vi "Compiled.Get Monitor Tool Settings.vi"(8 "error in (no error)":errorcluster, 9 "Database Ref":refnum<k21>, 11 "Addon Ref":T1 format="%.0x") -> (0 "error out":errorcluster, 2 "MonitorToolSettings":T2 {"Command Refs"."Response Refs"."Block Data Refs" format="%.0x"; "Command Refs"."Command Refs"."Block Data Refs"."Data Reference" format="%.0x"; "Data"."IncomingDataRefs"."Data Reference" format="%.0x"; "Data"."OutgoingDataRefs"."Data Reference" format="%.0x"; "Network"."Name" format="%.0x"}, 3 "Addon Ref out":T1 format="%.0x")   [LabVIEW 2015, in "J1939 Addon System Explorer.lvlib"]
uses:
  J1939 Addon System Explorer.lvlib
  <vilib>/NI Veristand/Custom Device API/Custom Device Item Ref.ctl
  Shared/Types/Compiled Monitor Tool Settings.ctl
  Shared/Types/Monitor Settings.ctl
  Shared/Types/Device Settings.ctl
  <vilib>/NI Veristand/Custom Device API/Block Data Reference.ctl
  <vilib>/NI Veristand/Custom Device API/Data Reference.ctl
  Shared/Types/Frame Settings.ctl
  Shared/Types/SysDef Command Settings.ctl
  <vilib>/NI Veristand/Custom Device Tools/Custom Device Utility Library/NI VeriStand - Search for Item by GUID.vi
  Shared/SubVIs/Constants.vi
  <vilib>/NI Veristand/Custom Device Tools/Custom Device Utility Library/Custom Device Utility Library.lvlib
  Shared/J1939 Addon Shared.lvlib
  <vilib>/NI VeriStand/Custom Device API/Custom Device API.lvlib
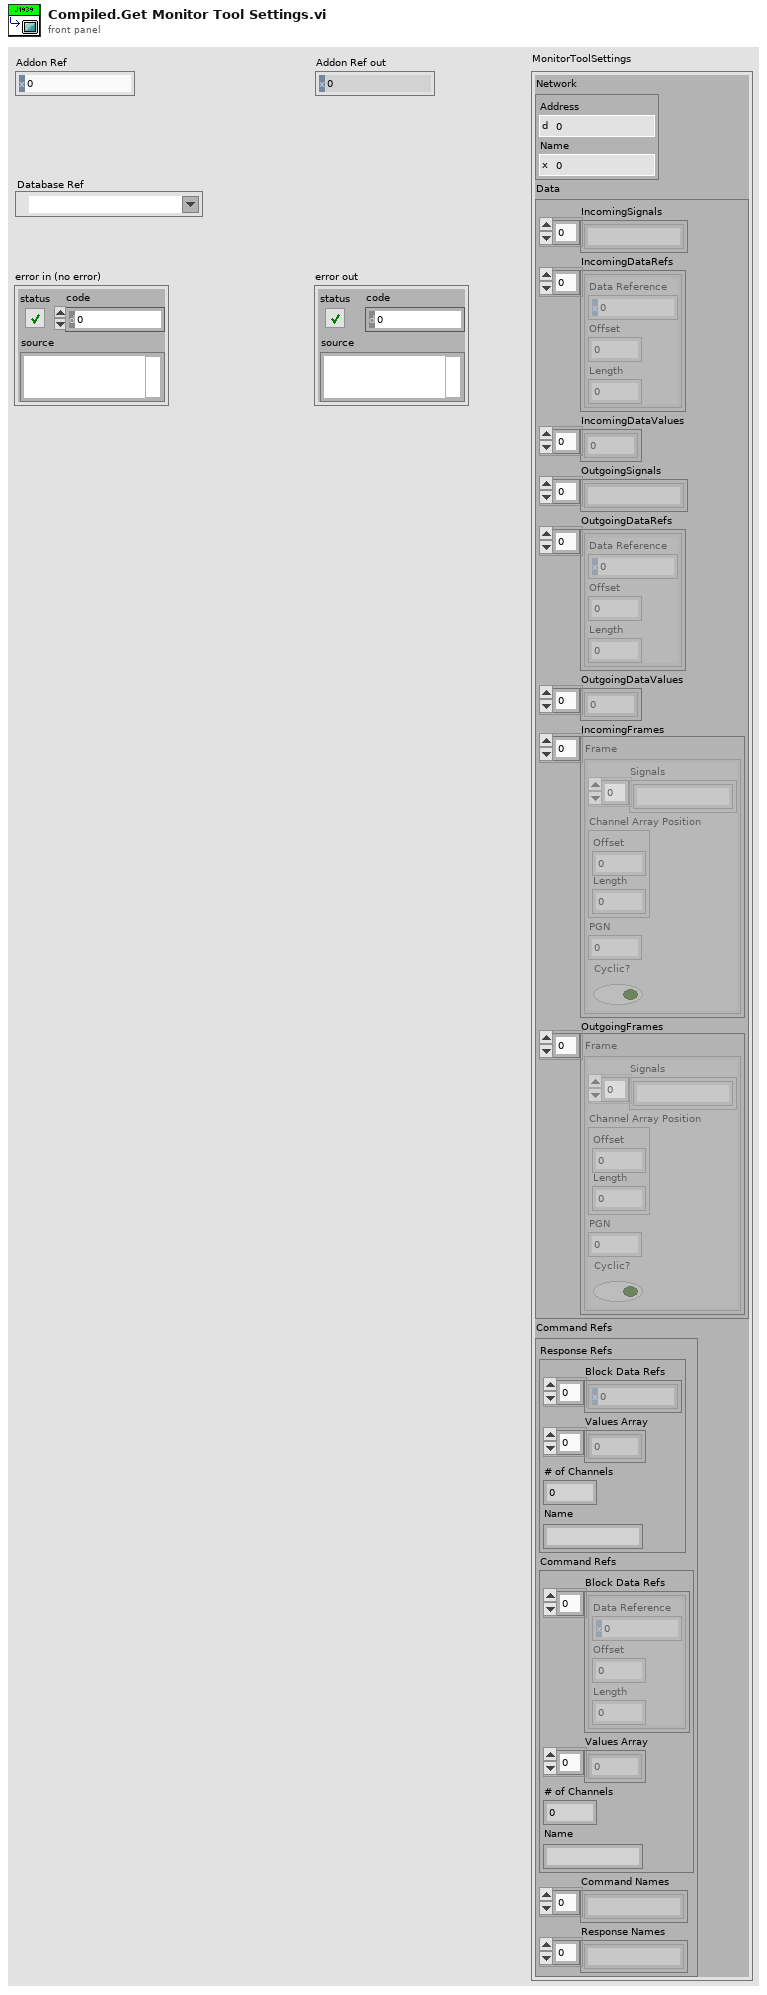
[diagram p1: front panel]
types:
  T1 = typedef "Custom Device API.lvlib/Custom Device Item Ref.ctl" = u64
  T2 = typedef "J1939 Addon Shared.lvlib/Compiled Monitor Tool Settings.ctl" = cluster{"Network":T3, "Data":T4, "Command Refs":T8}
  T3 = typedef "J1939 Addon Shared.lvlib/Monitor Settings.ctl" = cluster{"Address":u8, "Name":u64}
  T4 = typedef "J1939 Addon Shared.lvlib/Device Settings.ctl" = cluster{"IncomingSignals":string[], "IncomingDataRefs":T5[], "IncomingDataValues":dbl[], "OutgoingSignals":string[], "OutgoingDataRefs":T5[], "OutgoingDataValues":dbl[], "IncomingFrames":T7[], "OutgoingFrames":T7[]}
  T5 = typedef "Custom Device API.lvlib/Block Data Reference.ctl" = cluster{"Data Reference":T6, "Offset":u64, "Length":u64}
  T6 = typedef "Custom Device API.lvlib/Data Reference.ctl" = i32
  T7 = typedef "J1939 Addon Shared.lvlib/Frame Settings.ctl" = cluster{"Signals":string[], "Channel Array Position":cluster{"Offset":u32, "Length":u32}, "PGN":u32, "Cyclic?":bool}
  T8 = typedef "J1939 Addon Shared.lvlib/SysDef Command Settings.ctl" = cluster{"Response Refs":cluster{"Block Data Refs":T6[], "Values Array":dbl[], "# of Channels":u32, "Name":string}, "Command Refs":cluster{"Block Data Refs":T5[], "Values Array":dbl[], "# of Channels":u32, "Name":string}, "Command Names":string[], "Response Names":string[]}
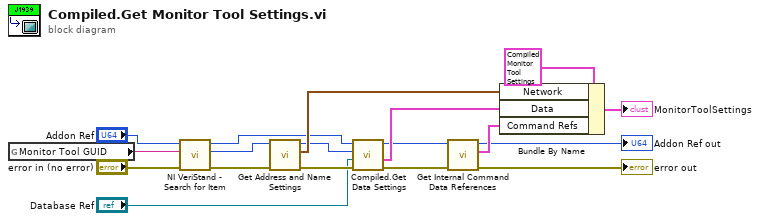
[diagram p0: block diagram]
diagram:
  n1 = global read "Constants.vi" "Monitor Tool GUID"() -> (w7:string)
  n2 = call-poly <vilib>:"NI VeriStand - Search for Item.vi"("error in"="error in (no error)", "Item GUID"=w7, "Section Ref in"="Addon Ref") -> ("error out"=w14:errorcluster, "Item Ref"=w15:T1, "Section Ref out"=w6:T1)  [unwired: 5 in, 1 out]
  n3 = call "Get Address and Name Settings.vi"("error in (no error)"=w14, "Node Ref"=w15) -> ("error out"=w12:errorcluster, "J1939 XNET Settings out"=w10:T3, "Node Ref out"=w5:T1)  [unwired: 7 in]
  n4 = call "Compiled.Get Data Settings.vi"("error in (no error)"=w12, "Database Ref"="Database Ref", "Node Ref in"=w5, "Addon Ref In"=w6) -> ("error out"=w9:errorcluster, "Node Data Refs"=w3:T4, "Addon Ref out"=w2:T1)  [unwired: 4 in, 1 out]
  n5 = call "Get Internal Command Data References.vi"("error in (no error)"=w9, "Addon Ref in"=w2) -> ("error out"=→"error out":errorcluster, "Internal Command Engine References"=w8:T8, "Addon Ref out"=→"Addon Ref out":T1)  [unwired: 7 in]
  n6 = Bundle By Name(cluster=T2 {"Network"={"Address"=0, "Name"=0}, "Data"={"IncomingSignals"=[], "IncomingDataRefs"=[], "IncomingDataValues"=[], "OutgoingSignals"=[], "OutgoingDataRefs"=[], "OutgoingDataValues"=[], "IncomingFrames"=[], "OutgoingFrames"=[]}, "Command Refs"={"Response Refs"={"Block Data Refs"=[], "Values Array"=[], "# of Channels"=0, "Name"=""}, "Command Refs"={"Block Data Refs"=[], "Values Array"=[], "# of Channels"=0, "Name"=""}, "Command Names"=[], "Response Names"=[]}} ("MonitorToolSettings"), "Network"=w10, "Data"=w3, "Command Refs"=w8) -> (→"MonitorToolSettings":T2)
